vi "Save Config.vi"(8 "error in (no error)":errorcluster, 11 "Coins":cluster{"Numeric":dbl, "Boolean Text":string}[](array[cluster])) -> (0 "error out":errorcluster)   [LabVIEW 2020, in "Config.lvlib"]
uses:
  <vilib>/Utility/xml.llb/Write to XML File(string).vi
  Config.lvlib
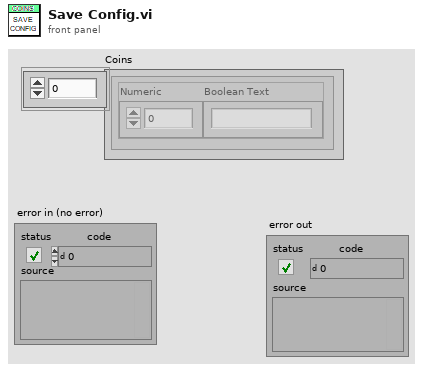
[diagram p1: front panel]
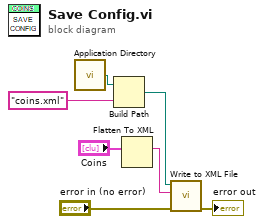
[diagram p0: block diagram]
diagram:
  n1 = call <vilib>:"Application Directory.vi"() -> ("Application Directory"=w7:path)
  n2 = Build Path(base path=w7, name or relative path="coins.xml") -> (appended path=w5:path)
  n3 = Flatten To XML(6:"Coins") -> (2:w4:string)
  n4 = call-poly <vilib>:"Write to XML File.vi"("error in (no error)"="error in (no error)", "XML Input"=w4, "XML File Path"=w5) -> ("error out"=→"error out":errorcluster)  [unwired: 6 in, 2 out]
